vi "day 14 task 2.vi"() -> ()   [LabVIEW 2019]
uses:
  48c75094-737f-452e-9833-d8298e23b8a0.vi
panel:
  out "tunnels":i16[][](array[numeric])
  out "x+y 2":i16[][](array[numeric])
  out "0, 2":i16[][](array[numeric])
  out "x*y":i32[][](array[numeric])
  out "x+y":u32[][](array[colorbox])
  out "0, 1":i16[][](array[numeric])
  out "Array 2":bool[][](array[boolean])
  out "Array":cluster{"x":i32, "y":i32}[](array[cluster])
  out "y of floor":i32
  out "no. units sand come to rest loop":u32
  out "no. units sand come to rest":u32
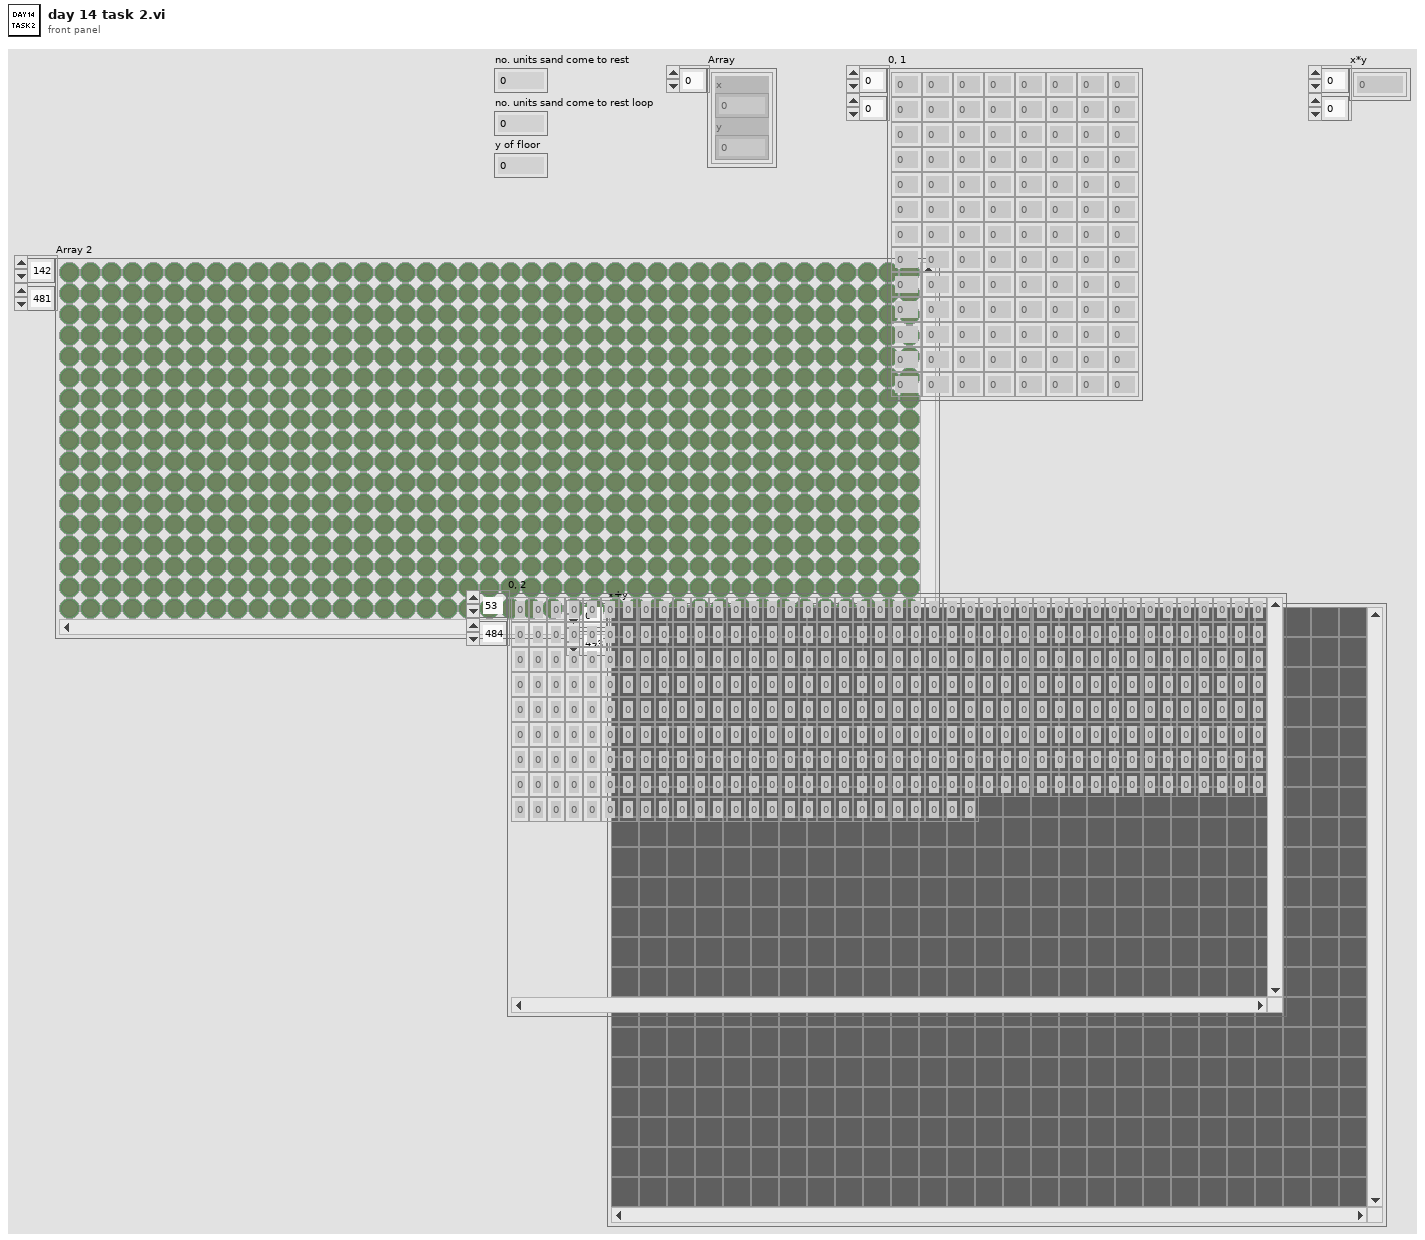
[diagram p1: front panel]
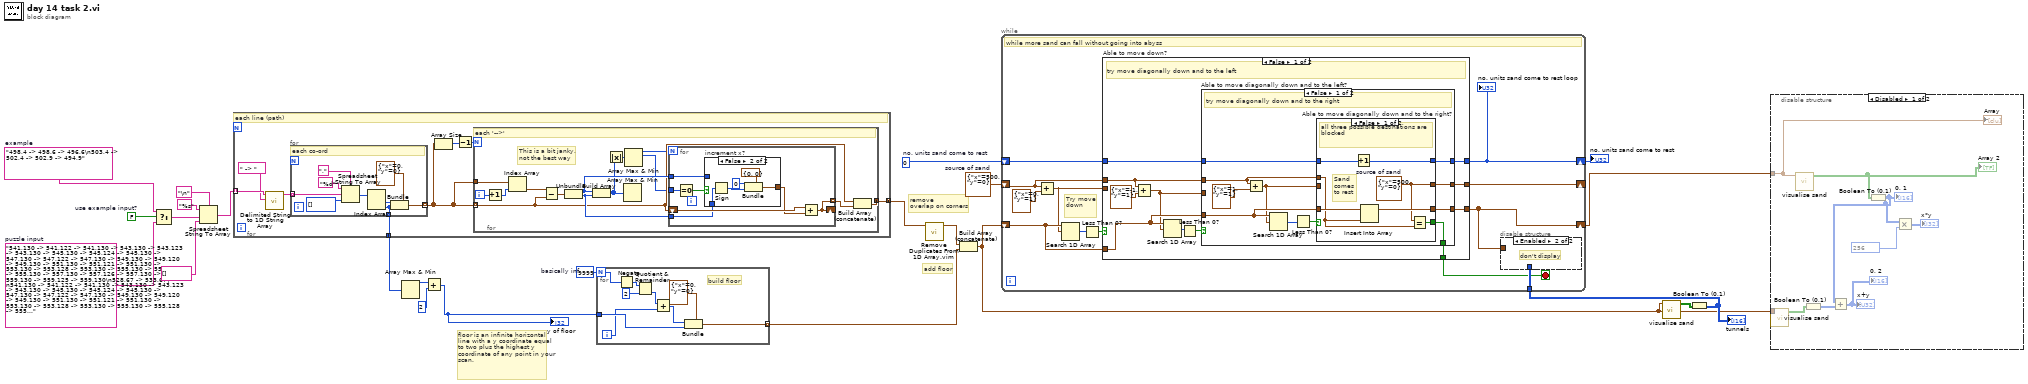
[diagram p0: block diagram]
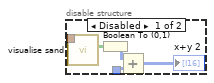
[diagram p2: hidden frame]
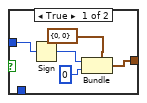
[diagram p7: hidden frame]
diagram:
  w10 = 9999  # basically inf
  w15 = cluster{"x":i32, "y":i32} {"x"=500, "y"=0}  # source of sand
  w16 = u32 0  # no. units sand come to rest
  w18 = FALSE  # use example input?
  w19 = "541,130 -> 541,122 -> 541,130 -> 543,130 -> 543,123 -> 543,130 -> 545,130 -> 545,124 -> 545,130 -> 547,130 -> 547,122 -> 547,130 -> 549,130 -> 549,120 -> 549,130 -> 551,130 -> 551,121 -> 551,130 -> 553,130 -> 553,128 -> 553,130 -> 555,130 -> 555,128 -> 555,130 -> 557,130 -> 557,126 -> 557,130 -> 559,130 -> 559,125 -> 559,130\n528,67 -> 533,67\n541,130 -> 541,122 -> 541,130 -> 543,130 -> 543,123 -> 543,130 -> 545,130 -> 545,124 -> 545,130 -> 547,130 -> 547,122 -> 547,130 -> 549,130 -> 549,120 -> 549,130 -> 551,130 -> 551,121 -> 551,130 -> 553,130 -> 553,128 -> 553,130 -> 555,130 -> 555,128 -> 555,130 -> 557,130 -> 557,126 -> 557,130 -> 559,130 -> 559,125 -> 559,130\n496,23 -> 496,16 -> 496,23 -> 498,23 -> 498,16 -> 498,23 -> 500,23 -> 500,17 -> 500,23 -> 502,23 -> 502,16 -> 502,23\n541,130 -> 541,122 -> 541,130 -> 543,130 -> 543,123 -> 543,130 -> 545,130 -> 545,124 -> 545,130 -> 547,130 -> 547,122 -> 547,130 -> 549,130 -> 549,120 -> 549,130 -> 551,130 -> 551,121 -> 551,130 -> 553,130 -> 553,128 -> 553,130 -> 555,130 -> 555,128 -> 555,130 -> 557,130 -> 557,126 -> 557,130 -> 559,130 -> 559,125 -> 559,130\n514,62 -> 519,62\n509,56 -> 514,56\n497,36 -> 497,30 -> 497,36 -> 499,36 -> 499,27 -> 499,36 -> 501,36 -> 501,33 -> 501,36 -> 503,36 -> 503,27 -> 503,36 -> 505,36 -> 505,28 -> 505,36 -> 507,36 -> 507,35 -> 507,36\n541,130 -> 541,122 -> 541,130 -> 543,130 -> 543,123 -> 543,130 -> 545,130 -> 545,124 -> 545,130 -> 547,130 -> 547,122 -> 547,130 -> 549,130 -> 549,120 -> 549,130 -> 551,130 -> 551,121 -> 551,130 -> 553,130 -> 553,128 -> 553,130 -> 555,130 -> 555,128 -> 555,130 -> 557,130 -> 557,126 -> 557,130 -> 559,130 -> 559,125 -> 559,130\n541,130 -> 541,122 -> 541,130 -> 543,130 -> 543,123 -> 543,130 -> 545,130 -> 545,124 -> 545,130 -> 547,130 -> 547,122 -> 547,130 -> 549,130 -> 549,120 -> 549,130 -> 551,130 -> 551,121 -> 551,130 -> 553,130 -> 553,128 -> 553,130 -> 555,130 -> 555,128 -> 555,130 -> 557,130 -> 557,126 -> 557,130 -> 559,130 -> 559,125 -> 559,130\n574,133 -> 574,137 -> 567,137 -> 567,141 -> 584,141 -> 584,137 -> 576,137 -> 576,133\n524,60 -> 529,60\n574,133 -> 574,137 -> 567,137 -> 567,141 -> 584,141 -> 584,137 -> 576,137 -> 576,133\n541,130 -> 541,122 -> 541,130 -> 543,130 -> 543,123 -> 543,130 -> 545,130 -> 545,124 -> 545,130 -> 547,130 -> 547,122 -> 547,130 -> 549,130 -> 549,120 -> 549,130 -> 551,130 -> 551,121 -> 551,130 -> 553,130 -> 553,128 -> 553,130 -> 555,130 -> 555,128 -> 555,130 -> 557,130 -> 557,126 -> 557,130 -> 559,130 -> 559,125 -> 559,130\n541,130 -> 541,122 -> 541,130 -> 543,130 -> 543,123 -> 543,130 -> 545,130 -> 545,124 -> 545,130 -> 547,130 -> 547,122 -> 547,130 -> 549,130 -> 549,120 -> 549,130 -> 551,130 -> 551,121 -> 551,130 -> 553,130 -> 553,128 -> 553,130 -> 555,130 -> 555,128 -> 555,130 -> 557,130 -> 557,126 -> 557,130 -> 559,130 -> 559,125 -> 559,130\n506,39 -> 506,43 -> 499,43 -> 499,51 -> 514,51 -> 514,43 -> 510,43 -> 510,39\n541,130 -> 541,122 -> 541,130 -> 543,130 -> 543,123 -> 543,130 -> 545,130 -> 545,124 -> 545,130 -> 547,130 -> 547,122 -> 547,130 -> 549,130 -> 549,120 -> 549,130 -> 551,130 -> 551,121 -> 551,130 -> 553,130 -> 553,128 -> 553,130 -> 555,130 -> 555,128 -> 555,130 -> 557,130 -> 557,126 -> 557,130 -> 559,130 -> 559,125 -> 559,130\n541,130 -> 541,122 -> 541,130 -> 543,130 -> 543,123 -> 543,130 -> 545,130 -> 545,124 -> 545,130 -> 547,130 -> 547,122 -> 547,130 -> 549,130 -> 549,120 -> 549,130 -> 551,130 -> 551,121 -> 551,130 -> 553,130 -> 553,128 -> 553,130 -> 555,130 -> 555,128 -> 555,130 -> 557,130 -> 557,126 -> 557,130 -> 559,130 -> 559,125 -> 559,130\n503,60 -> 508,60\n567,115 -> 571,115\n556,151 -> 556,153 -> 548,153 -> 548,157 -> 561,157 -> 561,153 -> 560,153 -> 560,151\n497,36 -> 497,30 -> 497,36 -> 499,36 -> 499,27 -> 499,36 -> 501,36 -> 501,33 -> 501,36 -> 503,36 -> 503,27 -> 503,36 -> 505,36 -> 505,28 -> 505,36 -> 507,36 -> 507,35 -> 507,36\n525,69 -> 530,69\n557,83 -> 557,85 -> 550,85 -> 550,89 -> 569,89 -> 569,85 -> 561,85 -> 561,83\n574,133 -> 574,137 -> 567,137 -> 567,141 -> 584,141 -> 584,137 -> 576,137 -> 576,133\n541,130 -> 541,122 -> 541,130 -> 543,130 -> 543,123 -> 543,130 -> 545,130 -> 545,124 -> 545,130 -> 547,130 -> 547,122 -> 547,130 -> 549,130 -> 549,120 -> 549,130 -> 551,130 -> 551,121 -> 551,130 -> 553,130 -> 553,128 -> 553,130 -> 555,130 -> 555,128 -> 555,130 -> 557,130 -> 557,126 -> 557,130 -> 559,130 -> 559,125 -> 559,130\n496,23 -> 496,16 -> 496,23 -> 498,23 -> 498,16 -> 498,23 -> 500,23 -> 500,17 -> 500,23 -> 502,23 -> 502,16 -> 502,23\n564,108 -> 564,107 -> 564,108 -> 566,108 -> 566,101 -> 566,108 -> 568,108 -> 568,100 -> 568,108\n496,23 -> 496,16 -> 496,23 -> 498,23 -> 498,16 -> 498,23 -> 500,23 -> 500,17 -> 500,23 -> 502,23 -> 502,16 -> 502,23\n556,151 -> 556,153 -> 548,153 -> 548,157 -> 561,157 -> 561,153 -> 560,153 -> 560,151\n541,130 -> 541,122 -> 541,130 -> 543,130 -> 543,123 -> 543,130 -> 545,130 -> 545,124 -> 545,130 -> 547,130 -> 547,122 -> 547,130 -> 549,130 -> 549,120 -> 549,130 -> 551,130 -> 551,121 -> 551,130 -> 553,130 -> 553,128 -> 553,130 -> 555,130 -> 555,128 -> 555,130 -> 557,130 -> 557,126 -> 557,130 -> 559,130 -> 559,125 -> 559,130\n497,36 -> 497,30 -> 497,36 -> 499,36 -> 499,27 -> 499,36 -> 501,36 -> 501,33 -> 501,36 -> 503,36 -> 503,27 -> 503,36 -> 505,36 -> 505,28 -> 505,36 -> 507,36 -> 507,35 -> 507,36\n556,151 -> 556,153 -> 548,153 -> 548,157 -> 561,157 -> 561,153 -> 560,153 -> 560,151\n561,115 -> 565,115\n564,144 -> 568,144\n497,36 -> 497,30 -> 497,36 -> 499,36 -> 499,27 -> 499,36 -> 501,36 -> 501,33 -> 501,36 -> 503,36 -> 503,27 -> 503,36 -> 505,36 -> 505,28 -> 505,36 -> 507,36 -> 507,35 -> 507,36\n541,130 -> 541,122 -> 541,130 -> 543,130 -> 543,123 -> 543,130 -> 545,130 -> 545,124 -> 545,130 -> 547,130 -> 547,122 -> 547,130 -> 549,130 -> 549,120 -> 549,130 -> 551,130 -> 551,121 -> 551,130 -> 553,130 -> 553,128 -> 553,130 -> 555,130 -> 555,128 -> 555,130 -> 557,130 -> 557,126 -> 557,130 -> 559,130 -> 559,125 -> 559,130\n497,36 -> 497,30 -> 497,36 -> 499,36 -> 499,27 -> 499,36 -> 501,36 -> 501,33 -> 501,36 -> 503,36 -> 503,27 -> 503,36 -> 505,36 -> 505,28 -> 505,36 -> 507,36 -> 507,35 -> 507,36\n556,151 -> 556,153 -> 548,153 -> 548,157 -> 561,157 -> 561,153 -> 560,153 -> 560,151\n557,83 -> 557,85 -> 550,85 -> 550,89 -> 569,89 -> 569,85 -> 561,85 -> 561,83\n496,23 -> 496,16 -> 496,23 -> 498,23 -> 498,16 -> 498,23 -> 500,23 -> 500,17 -> 500,23 -> 502,23 -> 502,16 -> 502,23\n567,146 -> 571,146\n531,65 -> 536,65\n528,62 -> 533,62\n541,130 -> 541,122 -> 541,130 -> 543,130 -> 543,123 -> 543,130 -> 545,130 -> 545,124 -> 545,130 -> 547,130 -> 547,122 -> 547,130 -> 549,130 -> 549,120 -> 549,130 -> 551,130 -> 551,121 -> 551,130 -> 553,130 -> 553,128 -> 553,130 -> 555,130 -> 555,128 -> 555,130 -> 557,130 -> 557,126 -> 557,130 -> 559,130 -> 559,125 -> 559,130\n541,130 -> 541,122 -> 541,130 -> 543,130 -> 543,123 -> 543,130 -> 545,130 -> 545,124 -> 545,130 -> 547,130 -> 547,122 -> 547,130 -> 549,130 -> 549,120 -> 549,130 -> 551,130 -> 551,121 -> 551,130 -> 553,130 -> 553,128 -> 553,130 -> 555,130 -> 555,128 -> 555,130 -> 557,130 -> 557,126 -> 557,130 -> 559,130 -> 559,125 -> 559,130\n574,133 -> 574,137 -> 567,137 -> 567,141 -> 584,141 -> 584,137 -> 576,137 -> 576,133\n568,95 -> 571,95 -> 571,94\n497,36 -> 497,30 -> 497,36 -> 499,36 -> 499,27 -> 499,36 -> 501,36 -> 501,33 -> 501,36 -> 503,36 -> 503,27 -> 503,36 -> 505,36 -> 505,28 -> 505,36 -> 507,36 -> 507,35 -> 507,36\n497,36 -> 497,30 -> 497,36 -> 499,36 -> 499,27 -> 499,36 -> 501,36 -> 501,33 -> 501,36 -> 503,36 -> 503,27 -> 503,36 -> 505,36 -> 505,28 -> 505,36 -> 507,36 -> 507,35 -> 507,36\n497,36 -> 497,30 -> 497,36 -> 499,36 -> 499,27 -> 499,36 -> 501,36 -> 501,33 -> 501,36 -> 503,36 -> 503,27 -> 503,36 -> 505,36 -> 505,28 -> 505,36 -> 507,36 -> 507,35 -> 507,36\n541,130 -> 541,122 -> 541,130 -> 543,130 -> 543,123 -> 543,130 -> 545,130 -> 545,124 -> 545,130 -> 547,130 -> 547,122 -> 547,130 -> 549,130 -> 549,120 -> 549,130 -> 551,130 -> 551,121 -> 551,130 -> 553,130 -> 553,128 -> 553,130 -> 555,130 -> 555,128 -> 555,130 -> 557,130 -> 557,126 -> 557,130 -> 559,130 -> 559,125 -> 559,130\n557,83 -> 557,85 -> 550,85 -> 550,89 -> 569,89 -> 569,85 -> 561,85 -> 561,83\n543,72 -> 543,73 -> 554,73 -> 554,72\n506,39 -> 506,43 -> 499,43 -> 499,51 -> 514,51 -> 514,43 -> 510,43 -> 510,39\n555,115 -> 559,115\n496,23 -> 496,16 -> 496,23 -> 498,23 -> 498,16 -> 498,23 -> 500,23 -> 500,17 -> 500,23 -> 502,23 -> 502,16 -> 502,23\n506,39 -> 506,43 -> 499,43 -> 499,51 -> 514,51 -> 514,43 -> 510,43 -> 510,39\n536,75 -> 536,76 -> 547,76 -> 547,75\n521,62 -> 526,62\n564,108 -> 564,107 -> 564,108 -> 566,108 -> 566,101 -> 566,108 -> 568,108 -> 568,100 -> 568,108\n574,133 -> 574,137 -> 567,137 -> 567,141 -> 584,141 -> 584,137 -> 576,137 -> 576,133\n516,56 -> 521,56\n564,108 -> 564,107 -> 564,108 -> 566,108 -> 566,101 -> 566,108 -> 568,108 -> 568,100 -> 568,108\n543,72 -> 543,73 -> 554,73 -> 554,72\n574,133 -> 574,137 -> 567,137 -> 567,141 -> 584,141 -> 584,137 -> 576,137 -> 576,133\n564,113 -> 568,113\n506,39 -> 506,43 -> 499,43 -> 499,51 -> 514,51 -> 514,43 -> 510,43 -> 510,39\n541,130 -> 541,122 -> 541,130 -> 543,130 -> 543,123 -> 543,130 -> 545,130 -> 545,124 -> 545,130 -> 547,130 -> 547,122 -> 547,130 -> 549,130 -> 549,120 -> 549,130 -> 551,130 -> 551,121 -> 551,130 -> 553,130 -> 553,128 -> 553,130 -> 555,130 -> 555,128 -> 555,130 -> 557,130 -> 557,126 -> 557,130 -> 559,130 -> 559,125 -> 559,130\n496,23 -> 496,16 -> 496,23 -> 498,23 -> 498,16 -> 498,23 -> 500,23 -> 500,17 -> 500,23 -> 502,23 -> 502,16 -> 502,23\n557,83 -> 557,85 -> 550,85 -> 550,89 -> 569,89 -> 569,85 -> 561,85 -> 561,83\n558,113 -> 562,113\n497,36 -> 497,30 -> 497,36 -> 499,36 -> 499,27 -> 499,36 -> 501,36 -> 501,33 -> 501,36 -> 503,36 -> 503,27 -> 503,36 -> 505,36 -> 505,28 -> 505,36 -> 507,36 -> 507,35 -> 507,36\n506,39 -> 506,43 -> 499,43 -> 499,51 -> 514,51 -> 514,43 -> 510,43 -> 510,39\n497,36 -> 497,30 -> 497,36 -> 499,36 -> 499,27 -> 499,36 -> 501,36 -> 501,33 -> 501,36 -> 503,36 -> 503,27 -> 503,36 -> 505,36 -> 505,28 -> 505,36 -> 507,36 -> 507,35 -> 507,36\n568,95 -> 571,95 -> 571,94\n497,36 -> 497,30 -> 497,36 -> 499,36 -> 499,27 -> 499,36 -> 501,36 -> 501,33 -> 501,36 -> 503,36 -> 503,27 -> 503,36 -> 505,36 -> 505,28 -> 505,36 -> 507,36 -> 507,35 -> 507,36\n510,60 -> 515,60\n497,36 -> 497,30 -> 497,36 -> 499,36 -> 499,27 -> 499,36 -> 501,36 -> 501,33 -> 501,36 -> 503,36 -> 503,27 -> 503,36 -> 505,36 -> 505,28 -> 505,36 -> 507,36 -> 507,35 -> 507,36\n557,83 -> 557,85 -> 550,85 -> 550,89 -> 569,89 -> 569,85 -> 561,85 -> 561,83\n570,117 -> 574,117\n497,36 -> 497,30 -> 497,36 -> 499,36 -> 499,27 -> 499,36 -> 501,36 -> 501,33 -> 501,36 -> 503,36 -> 503,27 -> 503,36 -> 505,36 -> 505,28 -> 505,36 -> 507,36 -> 507,35 -> 507,36\n507,62 -> 512,62\n541,130 -> 541,122 -> 541,130 -> 543,130 -> 543,123 -> 543,130 -> 545,130 -> 545,124 -> 545,130 -> 547,130 -> 547,122 -> 547,130 -> 549,130 -> 549,120 -> 549,130 -> 551,130 -> 551,121 -> 551,130 -> 553,130 -> 553,128 -> 553,130 -> 555,130 -> 555,128 -> 555,130 -> 557,130 -> 557,126 -> 557,130 -> 559,130 -> 559,125 -> 559,130\n556,151 -> 556,153 -> 548,153 -> 548,157 -> 561,157 -> 561,153 -> 560,153 -> 560,151\n564,108 -> 564,107 -> 564,108 -> 566,108 -> 566,101 -> 566,108 -> 568,108 -> 568,100 -> 568,108\n541,130 -> 541,122 -> 541,130 -> 543,130 -> 543,123 -> 543,130 -> 545,130 -> 545,124 -> 545,130 -> 547,130 -> 547,122 -> 547,130 -> 549,130 -> 549,120 -> 549,130 -> 551,130 -> 551,121 -> 551,130 -> 553,130 -> 553,128 -> 553,130 -> 555,130 -> 555,128 -> 555,130 -> 557,130 -> 557,126 -> 557,130 -> 559,130 -> 559,125 -> 559,130\n506,39 -> 506,43 -> 499,43 -> 499,51 -> 514,51 -> 514,43 -> 510,43 -> 510,39\n564,108 -> 564,107 -> 564,108 -> 566,108 -> 566,101 -> 566,108 -> 568,108 -> 568,100 -> 568,108\n497,36 -> 497,30 -> 497,36 -> 499,36 -> 499,27 -> 499,36 -> 501,36 -> 501,33 -> 501,36 -> 503,36 -> 503,27 -> 503,36 -> 505,36 -> 505,28 -> 505,36 -> 507,36 -> 507,35 -> 507,36\n561,111 -> 565,111\n541,130 -> 541,122 -> 541,130 -> 543,130 -> 543,123 -> 543,130 -> 545,130 -> 545,124 -> 545,130 -> 547,130 -> 547,122 -> 547,130 -> 549,130 -> 549,120 -> 549,130 -> 551,130 -> 551,121 -> 551,130 -> 553,130 -> 553,128 -> 553,130 -> 555,130 -> 555,128 -> 555,130 -> 557,130 -> 557,126 -> 557,130 -> 559,130 -> 559,125 -> 559,130\n541,130 -> 541,122 -> 541,130 -> 543,130 -> 543,123 -> 543,130 -> 545,130 -> 545,124 -> 545,130 -> 547,130 -> 547,122 -> 547,130 -> 549,130 -> 549,120 -> 549,130 -> 551,130 -> 551,121 -> 551,130 -> 553,130 -> 553,128 -> 553,130 -> 555,130 -> 555,128 -> 555,130 -> 557,130 -> 557,126 -> 557,130 -> 559,130 -> 559,125 -> 559,130\n541,130 -> 541,122 -> 541,130 -> 543,130 -> 543,123 -> 543,130 -> 545,130 -> 545,124 -> 545,130 -> 547,130 -> 547,122 -> 547,130 -> 549,130 -> 549,120 -> 549,130 -> 551,130 -> 551,121 -> 551,130 -> 553,130 -> 553,128 -> 553,130 -> 555,130 -> 555,128 -> 555,130 -> 557,130 -> 557,126 -> 557,130 -> 559,130 -> 559,125 -> 559,130\n496,23 -> 496,16 -> 496,23 -> 498,23 -> 498,16 -> 498,23 -> 500,23 -> 500,17 -> 500,23 -> 502,23 -> 502,16 -> 502,23\n558,148 -> 562,148\n513,58 -> 518,58\n564,108 -> 564,107 -> 564,108 -> 566,108 -> 566,101 -> 566,108 -> 568,108 -> 568,100 -> 568,108\n558,117 -> 562,117\n557,83 -> 557,85 -> 550,85 -> 550,89 -> 569,89 -> 569,85 -> 561,85 -> 561,83\n546,79 -> 546,80 -> 558,80\n541,130 -> 541,122 -> 541,130 -> 543,130 -> 543,123 -> 543,130 -> 545,130 -> 545,124 -> 545,130 -> 547,130 -> 547,122 -> 547,130 -> 549,130 -> 549,120 -> 549,130 -> 551,130 -> 551,121 -> 551,130 -> 553,130 -> 553,128 -> 553,130 -> 555,130 -> 555,128 -> 555,130 -> 557,130 -> 557,126 -> 557,130 -> 559,130 -> 559,125 -> 559,130\n541,130 -> 541,122 -> 541,130 -> 543,130 -> 543,123 -> 543,130 -> 545,130 -> 545,124 -> 545,130 -> 547,130 -> 547,122 -> 547,130 -> 549,130 -> 549,120 -> 549,130 -> 551,130 -> 551,121 -> 551,130 -> 553,130 -> 553,128 -> 553,130 -> 555,130 -> 555,128 -> 555,130 -> 557,130 -> 557,126 -> 557,130 -> 559,130 -> 559,125 -> 559,130\n536,75 -> 536,76 -> 547,76 -> 547,75\n500,62 -> 505,62\n506,39 -> 506,43 -> 499,43 -> 499,51 -> 514,51 -> 514,43 -> 510,43 -> 510,39\n556,151 -> 556,153 -> 548,153 -> 548,157 -> 561,157 -> 561,153 -> 560,153 -> 560,151\n520,58 -> 525,58\n535,67 -> 540,67\n574,133 -> 574,137 -> 567,137 -> 567,141 -> 584,141 -> 584,137 -> 576,137 -> 576,133\n497,36 -> 497,30 -> 497,36 -> 499,36 -> 499,27 -> 499,36 -> 501,36 -> 501,33 -> 501,36 -> 503,36 -> 503,27 -> 503,36 -> 505,36 -> 505,28 -> 505,36 -> 507,36 -> 507,35 -> 507,36\n541,130 -> 541,122 -> 541,130 -> 543,130 -> 543,123 -> 543,130 -> 545,130 -> 545,124 -> 545,130 -> 547,130 -> 547,122 -> 547,130 -> 549,130 -> 549,120 -> 549,130 -> 551,130 -> 551,121 -> 551,130 -> 553,130 -> 553,128 -> 553,130 -> 555,130 -> 555,128 -> 555,130 -> 557,130 -> 557,126 -> 557,130 -> 559,130 -> 559,125 -> 559,130\n546,79 -> 546,80 -> 558,80\n564,108 -> 564,107 -> 564,108 -> 566,108 -> 566,101 -> 566,108 -> 568,108 -> 568,100 -> 568,108\n543,72 -> 543,73 -> 554,73 -> 554,72\n564,117 -> 568,117\n497,36 -> 497,30 -> 497,36 -> 499,36 -> 499,27 -> 499,36 -> 501,36 -> 501,33 -> 501,36 -> 503,36 -> 503,27 -> 503,36 -> 505,36 -> 505,28 -> 505,36 -> 507,36 -> 507,35 -> 507,36\n497,36 -> 497,30 -> 497,36 -> 499,36 -> 499,27 -> 499,36 -> 501,36 -> 501,33 -> 501,36 -> 503,36 -> 503,27 -> 503,36 -> 505,36 -> 505,28 -> 505,36 -> 507,36 -> 507,35 -> 507,36\n536,75 -> 536,76 -> 547,76 -> 547,75\n557,83 -> 557,85 -> 550,85 -> 550,89 -> 569,89 -> 569,85 -> 561,85 -> 561,83\n496,23 -> 496,16 -> 496,23 -> 498,23 -> 498,16 -> 498,23 -> 500,23 -> 500,17 -> 500,23 -> 502,23 -> 502,16 -> 502,23\n541,130 -> 541,122 -> 541,130 -> 543,130 -> 543,123 -> 543,130 -> 545,130 -> 545,124 -> 545,130 -> 547,130 -> 547,122 -> 547,130 -> 549,130 -> 549,120 -> 549,130 -> 551,130 -> 551,121 -> 551,130 -> 553,130 -> 553,128 -> 553,130 -> 555,130 -> 555,128 -> 555,130 -> 557,130 -> 557,126 -> 557,130 -> 559,130 -> 559,125 -> 559,130\n539,69 -> 544,69\n552,117 -> 556,117\n556,151 -> 556,153 -> 548,153 -> 548,157 -> 561,157 -> 561,153 -> 560,153 -> 560,151\n496,23 -> 496,16 -> 496,23 -> 498,23 -> 498,16 -> 498,23 -> 500,23 -> 500,17 -> 500,23 -> 502,23 -> 502,16 -> 502,23\n561,146 -> 565,146\n570,148 -> 574,148\n496,23 -> 496,16 -> 496,23 -> 498,23 -> 498,16 -> 498,23 -> 500,23 -> 500,17 -> 500,23 -> 502,23 -> 502,16 -> 502,23\n496,23 -> 496,16 -> 496,23 -> 498,23 -> 498,16 -> 498,23 -> 500,23 -> 500,17 -> 500,23 -> 502,23 -> 502,16 -> 502,23\n532,69 -> 537,69\n564,108 -> 564,107 -> 564,108 -> 566,108 -> 566,101 -> 566,108 -> 568,108 -> 568,100 -> 568,108\n512,54 -> 517,54\n541,130 -> 541,122 -> 541,130 -> 543,130 -> 543,123 -> 543,130 -> 545,130 -> 545,124 -> 545,130 -> 547,130 -> 547,122 -> 547,130 -> 549,130 -> 549,120 -> 549,130 -> 551,130 -> 551,121 -> 551,130 -> 553,130 -> 553,128 -> 553,130 -> 555,130 -> 555,128 -> 555,130 -> 557,130 -> 557,126 -> 557,130 -> 559,130 -> 559,125 -> 559,130\n541,130 -> 541,122 -> 541,130 -> 543,130 -> 543,123 -> 543,130 -> 545,130 -> 545,124 -> 545,130 -> 547,130 -> 547,122 -> 547,130 -> 549,130 -> 549,120 -> 549,130 -> 551,130 -> 551,121 -> 551,130 -> 553,130 -> 553,128 -> 553,130 -> 555,130 -> 555,128 -> 555,130 -> 557,130 -> 557,126 -> 557,130 -> 559,130 -> 559,125 -> 559,130\n517,60 -> 522,60\n564,148 -> 568,148\n506,58 -> 511,58\n541,130 -> 541,122 -> 541,130 -> 543,130 -> 543,123 -> 543,130 -> 545,130 -> 545,124 -> 545,130 -> 547,130 -> 547,122 -> 547,130 -> 549,130 -> 549,120 -> 549,130 -> 551,130 -> 551,121 -> 551,130 -> 553,130 -> 553,128 -> 553,130 -> 555,130 -> 555,128 -> 555,130 -> 557,130 -> 557,126 -> 557,130 -> 559,130 -> 559,125 -> 559,130\n541,130 -> 541,122 -> 541,130 -> 543,130 -> 543,123 -> 543,130 -> 545,130 -> 545,124 -> 545,130 -> 547,130 -> 547,122 -> 547,130 -> 549,130 -> 549,120 -> 549,130 -> 551,130 -> 551,121 -> 551,130 -> 553,130 -> 553,128 -> 553,130 -> 555,130 -> 555,128 -> 555,130 -> 557,130 -> 557,126 -> 557,130 -> 559,130 -> 559,125 -> 559,130"  # puzzle input
  w20 = "498,4 -> 498,6 -> 496,6\n503,4 -> 502,4 -> 502,9 -> 494,9"  # example
  # "add floor"
  # "floor is an infinite horizontal line with a y coordinate equal to two plus the highest y coordinate of any point in your scan."
  # "remove\noverlap on corners"
  n1 = Select(t=w20, s=w18, f=w19) -> (s? t:f=w17:string)
  n2 = Spreadsheet String To Array(delimiter (Tab)="\n", format string="%s", spreadsheet string=w17, array type (2D Dbl)=string[] []) -> (array=w4:string[])
  n3 = for {
    tunnel: w4 -> [w31] mode=indexing
    tunnel: [w25] -> w2 mode=concatenating
    tunnel: [w24] -> w3 mode=concatenating
    # "each line (path)"
    n4 = call <vilib>:"Delimited String to 1D String Array.vi"("delimiter"=" -> ", "delimited string"=w31) -> ("string array"=w29:string[])  [unwired: 9 in]
    n5 = for {
      tunnel: w29 -> [w68] mode=indexing
      tunnel: [w64] -> w26 mode=indexing
      tunnel: [w63] -> w24 mode=indexing
      # "each co-ord"
      n6 = Spreadsheet String To Array(delimiter (Tab)=",", format string="%d", spreadsheet string=w68, array type (2D Dbl)=i32[] []) -> (array=w67:i32[])
      n7 = Index Array(array=w67) -> (element #1=w66:i32, element #2=w63:i32)  [unwired: 2 in]
      n8 = Bundle(cluster=cluster{"x":i32, "y":i32} {"x"=0, "y"=0}, "x"=w66, "y"=w63) -> (w64:cluster{"x":i32, "y":i32})
    }
    n9 = Array Size(array=w26) -> (size(s)=w27:i32)
    n10 = Decrement(x=w27) -> (x-1=w28:i32)
    n11 = for {
      N: w28 -> [_]
      tunnel: w26 -> [w37] mode=indexing
      tunnel: w26 -> [w45]
      tunnel: [w38] -> w25 mode=concatenating
      i -> [w44]
      # "This is a bit janky, \nnot the best way"
      # "each '-->'"
      n12 = Increment(x=w44) -> (x+1=w43:i32)
      n13 = Index Array(array=w45, index=w43) -> (element=w39:cluster{"x":i32, "y":i32})
      n14 = Subtract(x=w39, y=w37) -> (x-y=w42:cluster{"x":i32, "y":i32})
      n15 = Unbundle(w42) -> ("x"=w41:i32, "y"=w40:i32)
      n16 = Build Array(w41, w40) -> (w35:i32[])
      n17 = Absolute Value(x=w35) -> (abs(x)=w34:i32[])
      n18 = Array Max & Min(array=w35) -> ()  [unwired: 4 out]
      n19 = Array Max & Min(array=w34) -> (max value=w33:i32, max index (indices)=w32:i32)  [unwired: 2 out]
      n20 = for {
        N: w33 -> [_]
        tunnel: w32 -> [w52]
        tunnel: w41 -> [w47]
        shift-right: [w48] -> _
        shift-left: w37 -> [w51]
        tunnel: [w48] -> w36 mode=indexing
        tunnel: w40 -> [w46]
        n21 = Equal To 0?(x=w52) -> (x = 0?=w49:bool)
        n22 = case "increment x?" shown="False" w49 {
          tunnel: [w55 w61] -> w50
          tunnel: w47 -> [w54 _]
          tunnel: w46 -> [_ w58]
          frame True {
            n23 = Sign(1:w54) -> (0:w53:i32)
            n24 = Bundle(cluster=cluster{"x":i32, "y":i32} {"x"=0, "y"=0}, "x"=w53, "y"=0) -> (w55:cluster{"x":i32, "y":i32})
          }
          frame False {
            n25 = Sign(1:w58) -> (0:w59:i32)
            n26 = Bundle(cluster=cluster{"x":i32, "y":i32} {"x"=0, "y"=0}, "x"=0 ("y"), "y"=w59) -> (w61:cluster{"x":i32, "y":i32})
          }
        }
        n27 = Add(x=w51, y=w50) -> (x+y=w48:cluster{"x":i32, "y":i32})
      }
      n28 = Build Array (concatenate)(w37, w36) -> (w38:cluster{"x":i32, "y":i32}[])
    }
  }
  n29 = Array Max & Min(array=w3) -> (max value=w13:i32)  [unwired: 3 out]
  n30 = Add(x=w13, y=2) -> (x+y=w11:i32)
  "y of floor" <- w11
  n31 = for {
    N: w10 -> [w78]
    tunnel: w11 -> [w79]
    tunnel: [w72] -> w8 mode=indexing
    i -> [w74]
    # "build floor"
    n32 = Negate(x=w78) -> (-x=w77:i32)
    n33 = Quotient & Remainder(x=w77, y=2) -> (floor(x/y)=w75:i32)  [unwired: 1 out]
    n34 = Add(x=w75, y=w74) -> (x+y=w73:i32)
    n35 = Bundle(cluster=cluster{"x":i32, "y":i32} {"x"=0, "y"=0}, "x"=w73, "y"=w79) -> (w72:cluster{"x":i32, "y":i32})
  }
  n36 = call "Remove Duplicates From 1D Array.vim"("array"=w2) -> ("array with duplicates removed"=w9:cluster{"x":i32, "y":i32}[])  [unwired: 10 in]
  n37 = Build Array (concatenate)(w9, w8) -> (w5:cluster{"x":i32, "y":i32}[])
  n38 = call "visualise sand.vi"("Array in"=w5) -> ("Array out"=w7:bool[][])  [unwired: 10 in]
  n39 = Boolean To (0,1)(Boolean=w7) -> (0, 1=w6:i16[][])
  "tunnels" <- w6
  n40 = while {
    shift-right: [w85] -> _
    shift-left: w15 -> [w88]
    shift-right: [w84] -> w14
    shift-left: w16 -> [w89]
    shift-right: [w83] -> w1
    shift-left: w5 -> [w87]
    tunnel: w6 -> [w82]
    stop <- w81 stop-if-true
    # "Try move down"
    # "while more sand can fall without going into abyss"
    n41 = Add(x=w88, y=cluster{"x":i32, "y":i32} {"x"=0, "y"=1} ("source of sand")) -> (x+y=w86:cluster{"x":i32, "y":i32})
    n42 = Search 1D Array(1D array=w87, element=w86) -> (index of element=w91:i32)  [unwired: 1 in]
    n43 = Less Than 0?(x=w91) -> (x < 0?=w90:bool)
    n44 = case "Able to move down?" shown="False" w90 {
      tunnel: w89 -> [w103 w135]
      tunnel: w88 -> [w104 _]
      tunnel: w87 -> [w105 w133]
      tunnel: [w102 w135] -> w84
      tunnel: [w100 w134] -> w85
      tunnel: [w99 w133] -> w83
      tunnel: w86 -> [_ w134]
      tunnel: [w98 _] -> w81
      frame False {
        # "try move diagonally down and to the left"
        n45 = Add(x=w104, y=cluster{"x":i32, "y":i32} {"x"=-1, "y"=1} ("source of sand")) -> (x+y=w101:cluster{"x":i32, "y":i32})
        n46 = Search 1D Array(1D array=w105, element=w101) -> (index of element=w107:i32)  [unwired: 1 in]
        n47 = Less Than 0?(x=w107) -> (x < 0?=w106:bool)
        n48 = case "Able to move diagonally down and to the left?" shown="False" w106 {
          tunnel: w105 -> [w114 w130]
          tunnel: w104 -> [w113 _]
          tunnel: w103 -> [w116 w132]
          tunnel: [w115 w132] -> w102
          tunnel: w101 -> [_ w131]
          tunnel: [w111 w131] -> w100
          tunnel: [w112 w130] -> w99
          tunnel: [w109 _] -> w98
          frame False {
            # "try move diagonally down and to the right"
            n49 = Add(x=w113, y=cluster{"x":i32, "y":i32} {"x"=1, "y"=1} ("source of sand")) -> (x+y=w110:cluster{"x":i32, "y":i32})
            n50 = Search 1D Array(1D array=w114, element=w110) -> (index of element=w118:i32)  [unwired: 1 in]
            n51 = Less Than 0?(x=w118) -> (x < 0?=w117:bool)
            n52 = case "Able to move diagonally down and to the right?" shown="False" w117 {
              tunnel: w116 -> [w126 w127]
              tunnel: [w121 w127] -> w115
              tunnel: w114 -> [w125 w128]
              tunnel: w113 -> [w122 _]
              tunnel: [w124 w128] -> w112
              tunnel: [w120 w129] -> w111
              tunnel: w110 -> [_ w129]
              tunnel: [w123 _] -> w109
              frame False {
                w120 = cluster{"x":i32, "y":i32} {"x"=500, "y"=0}  # source of sand
                # "Sand comes to rest"
                # "all three possible destinations are blocked"
                n53 = Increment(x=w126) -> (x+1=w121:u32)
                n54 = Insert Into Array(array=w125, new element=w122) -> (w124:cluster{"x":i32, "y":i32}[])  [unwired: 1 in]
                n55 = Equal?(x=w120, y=w122) -> (x = y?=w123:bool)
              }
              frame True {
                # "make move"
              }
            }
          }
          frame True {
            # "use this position for next turn"
          }
        }
      }
      frame True {
        # "use this position for next turn"
      }
    }
    "no. units sand come to rest loop" <- w84
    n56 = disable-structure shown="Enabled" {
      disable-tunnel: w83 -> [w97 _]
      disable-tunnel: w82 -> [w96 _]
      frame Disabled {
        n57 = call "visualise sand.vi"("Array in"=w97) -> ("Array out"=w95:bool[][])  [unwired: 10 in]
        n58 = Boolean To (0,1)(Boolean=w95) -> (0, 1=w94:i16[][])
        n59 = Add(x=w94, y=w96) -> (x+y=→"x+y 2":i16[][])
      }
      frame Enabled {
        # "don't display"
      }
    }
  }
  "no. units sand come to rest" <- w14
  n60 = disable-structure shown="Disabled" {
    disable-tunnel: w5 -> [w137 _]
    disable-tunnel: w1 -> [w136 _]
    frame Disabled {
      n61 = call "visualise sand.vi"("Array in"=w137) -> ("Array out"=w142:bool[][])  [unwired: 10 in]
      n62 = call "visualise sand.vi"("Array in"=w136) -> ("Array out"=w144:bool[][])  [unwired: 10 in]
      "Array 2" <- w144
      n63 = Boolean To (0,1)(Boolean=w142) -> (0, 1=w143:i16[][])
      n64 = Boolean To (0,1)(Boolean=w144) -> (0, 1=w141:i16[][])
      "0, 1" <- w141
      n65 = Add(x=w141, y=w143) -> (x+y=→"x+y" →"0, 2":i16[][])
      n66 = Multiply(x=w141, y=u32 256) -> (x*y=→"x*y":u32[][])
      "Array" <- w136
    }
    frame Enabled {
    }
  }
